vi "Ex9.vi"() -> ()   [LabVIEW 2016]
panel:
  out "로컬 변수 사용하여 배열 만들기":dbl[](array[numeric])
  out "초기화된 배열":dbl[](array[numeric])
  out "While loop 사용 배열 만들기":dbl[](array[numeric])
  out "For loop 사용 배열 만들기":dbl[](array[numeric])
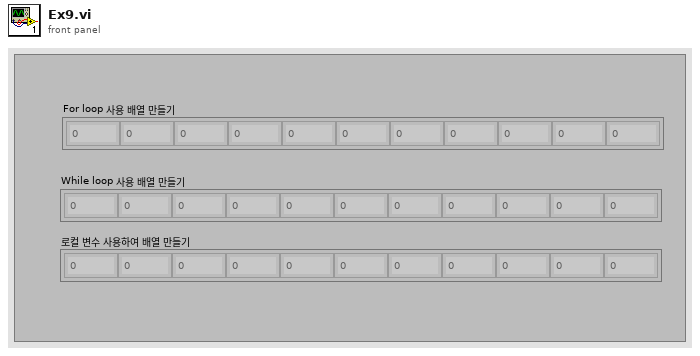
[diagram p1: front panel]
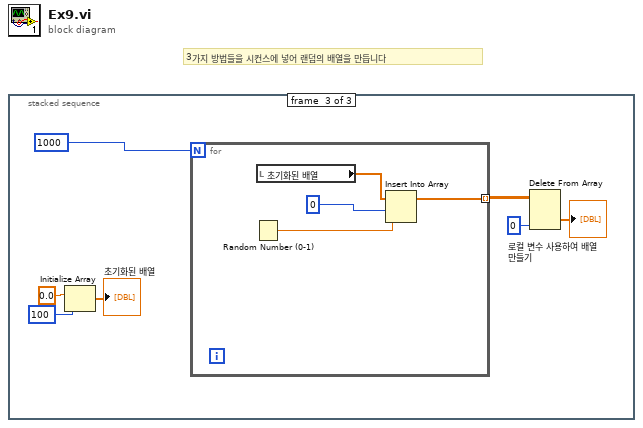
[diagram p0: block diagram]
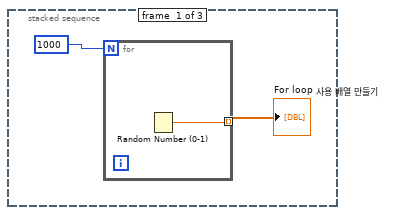
[diagram p2: hidden frame]
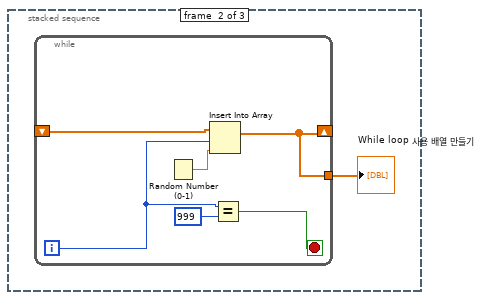
[diagram p3: hidden frame]
diagram:
  # "3가지 방법들을 시컨스에 넣어 랜덤의 배열을 만듭니다"
  n1 = stacked-sequence {
    frame #0 {
      n2 = for {
        N: 1000 -> [_]
        tunnel: [w3] -> w1 mode=indexing
        n3 = Random Number (0-1)() -> (number: 0 to 1=w3:dbl)
      }
      "For loop 사용 배열 만들기" <- w1
    }
    frame #1 {
      n4 = while {
        shift-right: [w5] -> _
        shift-left: _ -> [w10]
        tunnel: [w5] -> w4
        i -> [w8]
        stop <- w6 stop-if-true
        n5 = Random Number (0-1)() -> (number: 0 to 1=w9:dbl)
        n6 = Insert Into Array(array=w10, index=w8, new element=w9) -> (w5:dbl[])
        n7 = Equal?(x=w8, y=999) -> (x = y?=w6:bool)
      }
      "While loop 사용 배열 만들기" <- w4
    }
    frame #2 {
      n8 = Initialize Array(0.0 ("원소"), 100 ("차원 크기")) -> (→"초기화된 배열":dbl[])
      n9 = for {
        N: 1000 -> [_]
        tunnel: [w18] -> w13 mode=indexing
        n10 = Random Number (0-1)() -> (number: 0 to 1=w21:dbl)
        n11 = local read "초기화된 배열"() -> (w20:dbl[])
        n12 = Insert Into Array(array=w20, index=0 ("인덱스"), new element=w21) -> (w18:dbl[])
      }
      n13 = Delete From Array(array=w13, index (col)=0 ("비활성화된 인덱스 (열)")) -> (deleted portion=→"로컬 변수 사용하여 배열 만들기":dbl[])  [unwired: 2 in, 1 out]
    }
  }
